vi "Init Xnet Interfaces.vi"(8 "error in (no error)":errorcluster, 9 "Output Singals":refnum<k21>[](array[refnum]), 10 "Input Signals":refnum<k21>[](array[refnum]), 11 "Config In":refnum<class "J1939 configuration.lvclass">) -> (0 "error out":errorcluster, 1 "Output Session":refnum<k21>, 2 "Input Session":refnum<k21>, 3 "Config Out":refnum<class "J1939 configuration.lvclass">)   [LabVIEW 2015, in "J1939 runtime.lvclass"]
uses:
  J1939 runtime.lvclass
  configuration/J1939 configuration.lvclass
  configuration/J1939 configuration.lvclass/J1939 configuration.ctl
  configuration/Read XNET Settings.vi
  <vilib>/xnet/xnet.llb/XNET Create Session (Signal Input Single-point).vi
  J1939 Claim With Address.vi
  <vilib>/xnet/xnet.llb/XNET Create Session (Signal Output Single-point).vi
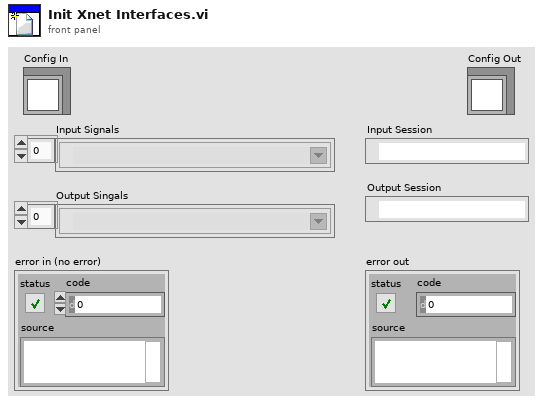
[diagram p1: front panel]
types:
  T1 = typedef "J1939 configuration.lvclass/XNET Settings.ctl" = cluster{"Select Interface":refnum<k21>, "Claim By Adress":bool, "Node Address":u8, "Node Name":u64}
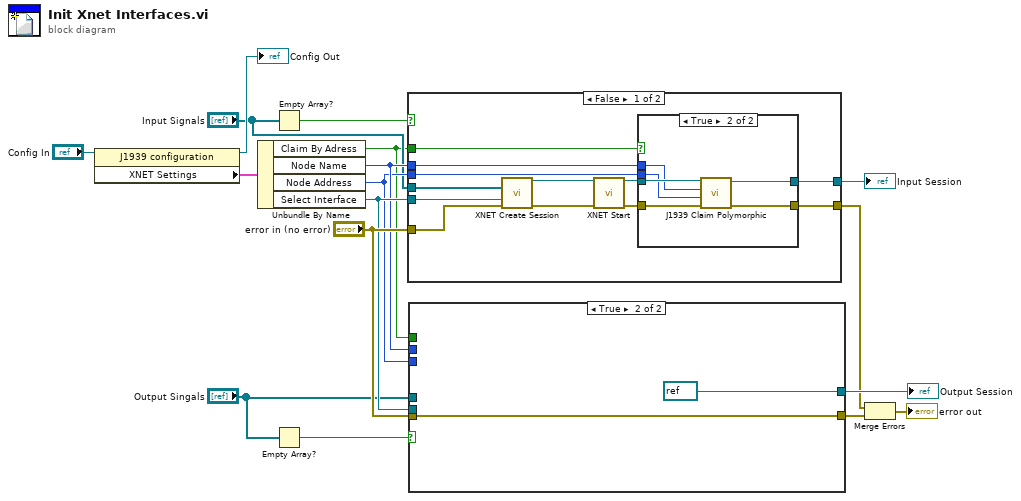
[diagram p0: block diagram]
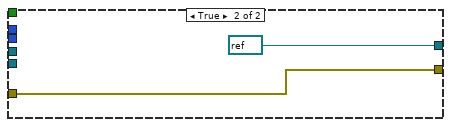
[diagram p3: hidden frame]
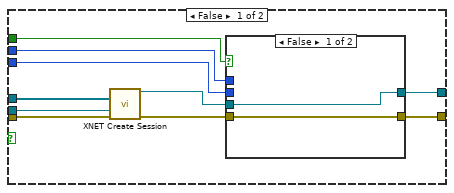
[diagram p4: hidden frame]
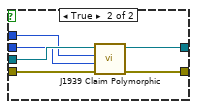
[diagram p5: hidden frame]
diagram:
  n1 = property class="J1939 configuration"(reference="Config In") -> (reference out=→"Config Out":refnum<class "J1939 configuration.lvclass">, "XNET Settings"=w9:T1)  [unwired: 1 in, 1 out]
  n2 = Unbundle By Name(w9) -> ("Claim By Adress"=w1:bool, "Node Name"=w7:u64, "Node Address"=w6:u8, "Select Interface"=w8:refnum<k21>)
  n3 = Empty Array?(array="Input Signals") -> (empty?=w4:bool)
  n4 = Empty Array?(array="Output Singals") -> (empty?=w3:bool)
  n5 = case shown="False" w4 {
    tunnel: "Input Signals" -> [w29 _]
    tunnel: "error in (no error)" -> [w28 w38]
    tunnel: [w24 w38] -> w13
    tunnel: [w23 refnum<k21> refnum ("XNET Session Out")] -> w12
    tunnel: w8 -> [w21 _]
    tunnel: w7 -> [w20 _]
    tunnel: w6 -> [w19 _]
    tunnel: w1 -> [w18 _]
    frame False {
      n6 = call-poly <vilib>:"XNET Create Session.vi"("signal list"=w29, "interface"=w21, "error in (no error)"=w28) -> ("session out"=w22:refnum<k21>, "error out"=w27:errorcluster)  [unwired: 11 out]
      n7 = call <vilib>:"XNET Start.vi"("session in"=w22, "error in (no error)"=w27) -> ("session out"=w25:refnum<k21>, "error out"=w26:errorcluster)  [unwired: 12 in]
      n8 = case shown="True" w18 {
        tunnel: w26 -> [w30 w37]
        tunnel: w25 -> [w31 w36]
        tunnel: [w30 w35] -> w24
        tunnel: [w31 w34] -> w23
        tunnel: w20 -> [_ w33]
        tunnel: w19 -> [_ w32]
        frame False {
        }
        frame True {
          n9 = call-poly "J1939 Claim Polymorphic.vi"("error in (no error)"=w37, "SAE J1939:Node Address"=w32, "SAE J1939:Node Name"=w33, "XNET Session"=w36) -> ("error out"=w35:errorcluster, "XNET Session Out"=w34:refnum<k21>)  [unwired: 5 in, 1 out]
        }
      }
    }
    frame True {
    }
  }
  "Input Session" <- w12
  n10 = case shown="True" w3 {
    tunnel: [w49 w59] -> w17
    tunnel: [w48 refnum<k21> refnum ("XNET Session Out")] -> w16
    tunnel: "Output Singals" -> [w47 _]
    tunnel: "error in (no error)" -> [w44 w59]
    tunnel: w8 -> [w43 _]
    tunnel: w7 -> [w42 _]
    tunnel: w6 -> [w41 _]
    tunnel: w1 -> [w40 _]
    frame False {
      n11 = call-poly <vilib>:"XNET Create Session.vi"("signal list"=w47, "interface"=w43, "error in (no error)"=w44) -> ("session out"=w45:refnum<k21>, "error out"=w46:errorcluster)  [unwired: 1 in, 10 out]
      n12 = case shown="False" w40 {
        tunnel: [w50 w57] -> w49
        tunnel: [w51 w56] -> w48
        tunnel: w46 -> [w50 w55]
        tunnel: w45 -> [w51 w54]
        tunnel: w42 -> [_ w53]
        tunnel: w41 -> [_ w52]
        frame False {
        }
        frame True {
          n13 = call-poly "J1939 Claim Polymorphic.vi"("error in (no error)"=w55, "SAE J1939:Node Address"=w52, "SAE J1939:Node Name"=w53, "XNET Session"=w54) -> ("error out"=w57:errorcluster, "XNET Session Out"=w56:refnum<k21>)  [unwired: 5 in, 1 out]
        }
      }
    }
    frame True {
    }
  }
  "Output Session" <- w16
  n14 = Merge Errors(w13, w17) -> (→"error out":errorcluster)
